vi "Copy From Panel to Private Data.vi"(6 "Add as Reference?":bool, 8 "error in (no error)":errorcluster, 9 "Text to Append (\" Ref\")":string=" Ref", 10 "GObjects in":refnum<vi>[](array[refnum]), 11 "Private Data Refs":T1) -> (0 "error out":errorcluster, 2 "Other GObjects":refnum<vi>[](array[refnum]), 3 "ControlReferenceConstants":refnum<vi>[](array[refnum]))   [LabVIEW 2020, in "Add to Private Data.lvlib"]
uses:
  Add to Private Data.lvlib
  Private Data Refs.ctl
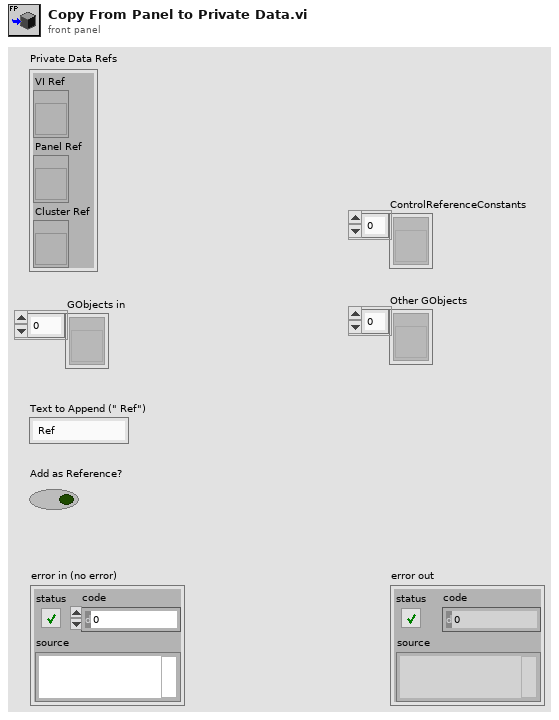
[diagram p1: front panel]
types:
  T1 = typedef "Add to Private Data.lvlib/Private Data Refs.ctl" = cluster{"VI Ref":refnum<vi>, "Panel Ref":refnum<vi>, "Cluster Ref":refnum<vi>}
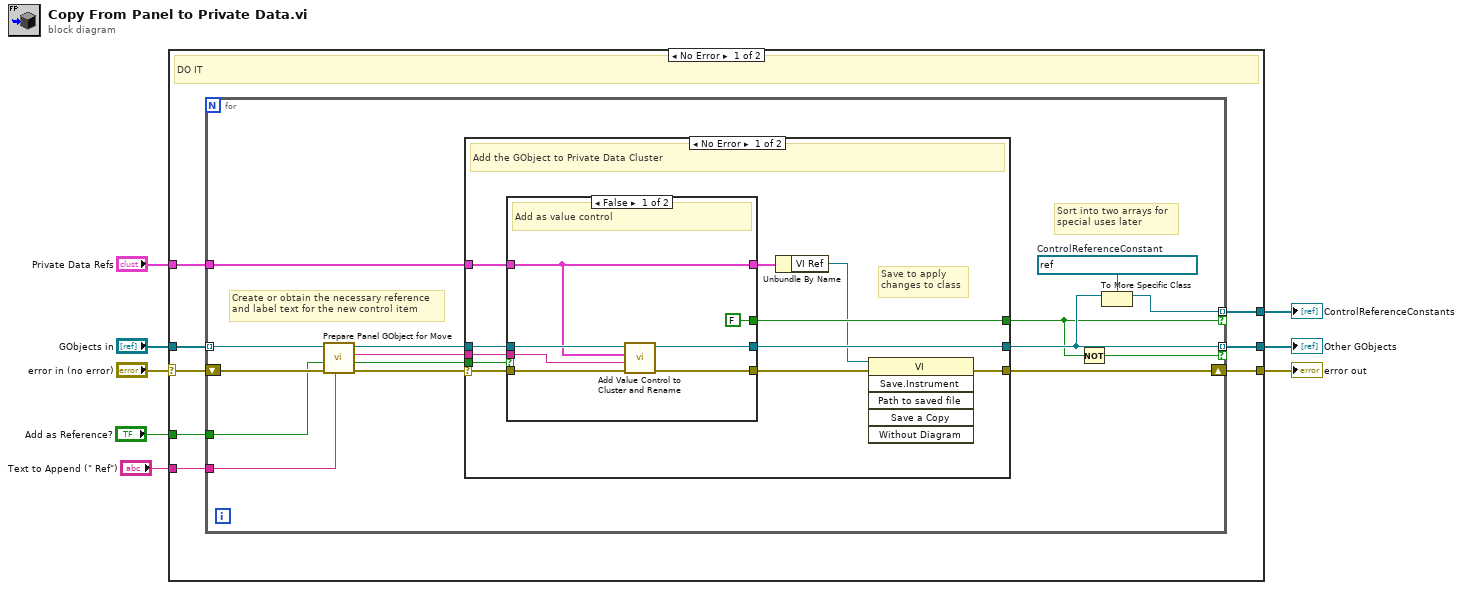
[diagram p0: block diagram]
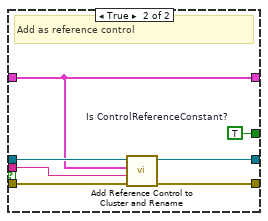
[diagram p2: hidden frame]
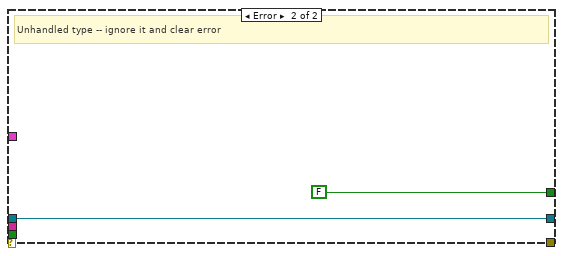
[diagram p3: hidden frame]
diagram:
  n1 = case shown="No Error" "error in (no error)" {
    selector: "error in (no error)" -> [w9 w59]
    tunnel: [w16 w59] -> w8
    tunnel: "GObjects in" -> [w15 w60]
    tunnel: "Text to Append (\" Ref\")" -> [w14 _]
    tunnel: "Private Data Refs" -> [w13 _]
    tunnel: "Add as Reference?" -> [w12 _]
    tunnel: [w11 w60] -> w3
    tunnel: [w10 _] -> w2
    frame No Error {
      # "DO IT"
      n2 = for {
        tunnel: w15 -> [w30] mode=indexing
        tunnel: w14 -> [w31]
        tunnel: w13 -> [w24]
        shift-right: [w23] -> w16
        shift-left: w9 -> [w29]
        tunnel: w12 -> [w22]
        tunnel: [w21] -> w11 mode=indexing if=w18
        tunnel: [w20] -> w10 mode=indexing if=w17
        w19 = refnum<vi> refnum  # ControlReferenceConstant
        # "Sort into two arrays for\nspecial uses later"
        # "Create or obtain the necessary reference\nand label text for the new control item"
        n3 = call "Prepare Panel GObject for Move.vi"("Reference Text to Append (\" Ref\")"=w31, "error in (no error)"=w29, "Add as Reference?"=w22, "GObject in"=w30) -> ("error out"=w28:errorcluster, "Updated Add as Reference?"=w26:bool, "Label.Text"=w25:string, "GObject out"=w27:refnum<vi>)  [unwired: 4 in]
        n4 = case shown="No Error" w28 {
          selector: w28 -> [w38 _]
          tunnel: [w34 _] -> w23
          tunnel: w24 -> [w41 _]
          tunnel: w27 -> [w40 w58]
          tunnel: w25 -> [w39 _]
          tunnel: w26 -> [w37 _]
          tunnel: [w36 w58] -> w21
          tunnel: [w35 FALSE ("Is ControlReferenceConstant?")] -> w17
          frame No Error {
            # "Save to apply\nchanges to class"
            # "Add the GObject to Private Data Cluster"
            n5 = case shown="False" w37 {
              tunnel: [w49 w55] -> w42
              tunnel: w40 -> [w46 w54]
              tunnel: w38 -> [w48 w56]
              tunnel: w41 -> [w43 w50]
              tunnel: w39 -> [w47 w53]
              tunnel: [w45 w52] -> w36
              tunnel: [FALSE w51] -> w35
              tunnel: [w43 w50] -> w33
              frame False {
                # "Add as value control"
                n6 = call "Add Value Control to Cluster and Rename.vi"("error in (no error)"=w48, "New Label.Text"=w47, "Private Data Refs"=w43, "GObject in"=w46) -> ("error out"=w49:errorcluster, "GObject out"=w45:refnum<vi>)  [unwired: 6 in]
              }
              frame True {
                w51 = TRUE  # Is ControlReferenceConstant?
                # "Add as reference control"
                n7 = call "Add Reference Control to Cluster and Rename.vi"("error in (no error)"=w56, "New Label.Text"=w53, "Private Data Refs"=w50, "GObject in"=w54) -> ("error out"=w55:errorcluster, "GObject out"=w52:refnum<vi>)  [unwired: 6 in]
              }
            }
            n8 = Unbundle By Name(w33) -> ("VI Ref"=w32:refnum<vi>)
            n9 = invoke class="VI" method="Save.Instrument"(reference=w32, error in=w42) -> (error out=w34:errorcluster)  [unwired: 4 in, 5 out]
          }
          frame Error {
            # "Unhandled type -- ignore it and clear error"
          }
        }
        n10 = Not(x=w17) -> (.not. x?=w18:bool)
        n11 = To More Specific Class(target class=w19, reference=w21) -> (specific class reference=w20:refnum<vi>)  [unwired: 1 in, 1 out]
      }
    }
    frame Error {
      # "Calling VI is probably not a member of a class. Regardless, do nothing."
    }
  }
  "error out" <- w8
  "Other GObjects" <- w3
  "ControlReferenceConstants" <- w2
